vi "Open Magnet Device.vi"(8 "error in (no error)":errorcluster, 10 "Device Identifier":T1="GRPZ", 11 "Mercury Reference In":T2) -> (0 "error out":errorcluster, 3 "Mercury Reference Out":T2)   [LabVIEW 2018, in "Mercury iXX.lvlib" / "Magnet.lvlib"]
doc: "Opens a reference to a device within the current Mercury instrument you are connected to.\n\nOpen System must be called before this function."
uses:
  Magnet.lvlib
  Mercury Reference.ctl
  Comms Transport Layer.ctl
  Query Dynamic Reference.ctl
  Identifier.ctl
  Mercury iXX.lvlib
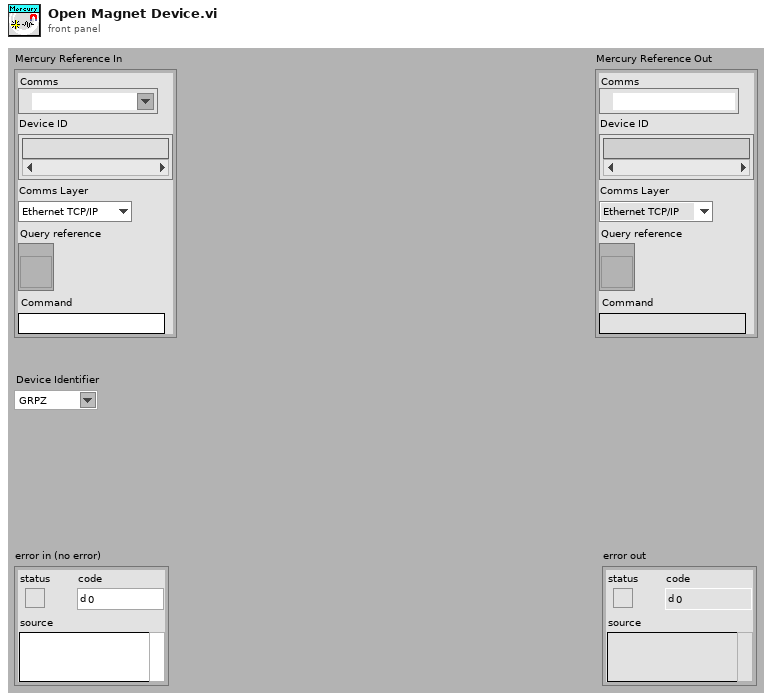
[diagram p1: front panel]
types:
  T1 = typedef "Mercury iXX.lvlib/Magnet.lvlib/Identifier.ctl" = string
  T2 = typedef "Mercury iXX.lvlib/Mercury Reference.ctl" = cluster{"Comms":refnum<visa-resource-name>, "Device ID":string[], "Comms Layer":T3, "Command":string, "Query reference":T4}
  T3 = typedef "Mercury iXX.lvlib/Comms Transport Layer.ctl" = enum16{"Ethernet TCP/IP", "USB", "ISOBus - RS-232", "GPIB"}
  T4 = typedef "Mercury iXX.lvlib/Query Dynamic Reference.ctl" = refnum<vi>
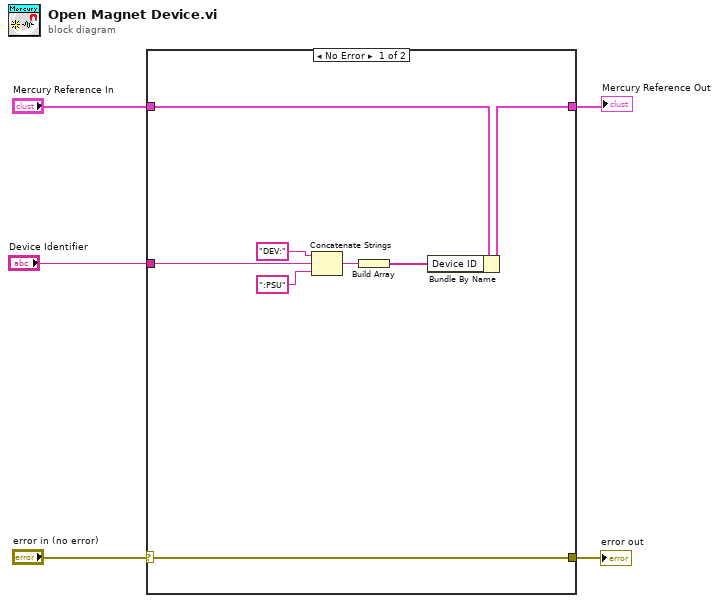
[diagram p0: block diagram]
diagram:
  n1 = case shown="No Error" "error in (no error)" {
    selector: "error in (no error)" -> [w11 w15]
    tunnel: "Mercury Reference In" -> [w13 w14]
    tunnel: [w12 w14] -> w4
    tunnel: [w11 w15] -> w2
    tunnel: "Device Identifier" -> [w10 _]
    frame No Error {
      n2 = Concatenate Strings("DEV:" ("element"), w10, ":PSU" ("element")) -> (w8:string)
      n3 = Build Array(w8) -> (w9:string[])
      n4 = Bundle By Name(cluster=w13, "Device ID"=w9) -> (w12:T2)
    }
    frame Error {
    }
  }
  "Mercury Reference Out" <- w4
  "error out" <- w2
